vi "GetParam.vi"(8 "error in (no error)":errorcluster caption="entrée d'erreur (pas d'erreur)", 11 "Friedman2.lvclass":refnum<class "Friedman2.lvclass">) -> (0 "error out":errorcluster caption="sortie d'erreur", 2 "make_friedman2":T1={"n_samples"=100, "noise"=0.0, "random_state"=-1, "Returns"="X"} {"random_state" min=-1; "n_samples" min=1}, 3 "Friedman2.lvclass":refnum<class "Friedman2.lvclass">)   [LabVIEW 2020, in "Friedman2.lvclass"]
doc: "Get Parameters"
uses:
  Friedman2.lvclass
  Friedman2.lvclass/Friedman2.ctl
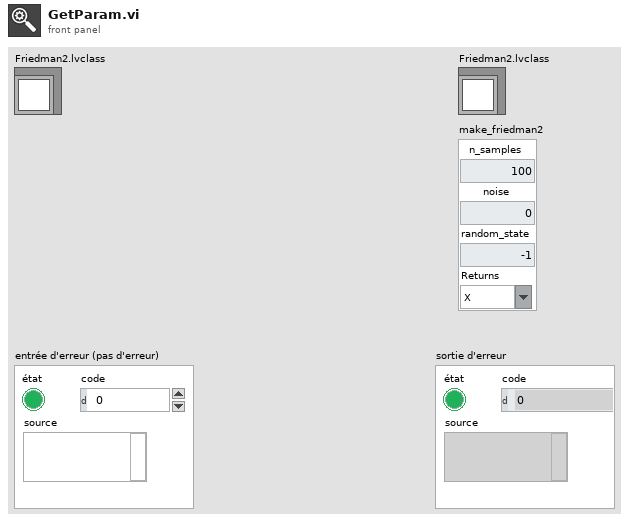
[diagram p1: front panel]
types:
  T1 = cluster{"n_samples":u32, "noise":dbl, "random_state":i32, "Returns":string}
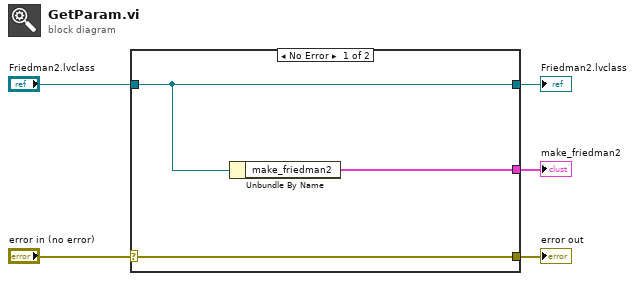
[diagram p0: block diagram]
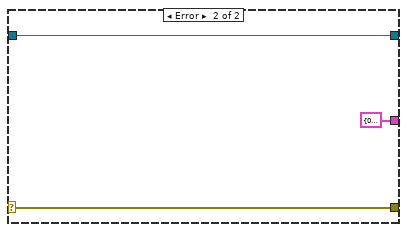
[diagram p2: hidden frame]
diagram:
  n1 = case shown="No Error" "error in (no error)" {
    selector: "error in (no error)" -> [w8 w10]
    tunnel: [w8 w10] -> w4
    tunnel: [w7 w11] -> w2
    tunnel: "Friedman2.lvclass" -> [w7 w11]
    tunnel: [w6 T1 {"n_samples"=0, "noise"=0.0, "random_state"=0, "Returns"=""} ("make_friedman2")] -> w1
    frame No Error {
      n2 = Unbundle By Name(w7) -> ("make_friedman2"=w6:T1)
    }
    frame Error {
    }
  }
  "error out" <- w4
  "Friedman2.lvclass" <- w2
  "make_friedman2" <- w1
